vi "Send Serial Command.vi"(7 "Listen for response (T)":bool=TRUE, 8 "error in (no error)":errorcluster, 10 "Command":string, 11 "VISA in":refnum<visa-resource-name>) -> (0 "error out":errorcluster, 2 "Response":string, 3 "VISA out":refnum<visa-resource-name>)   [LabVIEW 2017, in "Drivers.lvlib" / "ASI TG-1000.lvlib"]
doc: "Sends serial command to ASI controller, which should already be configured and initialized."
uses:
  ASI TG-1000.lvlib
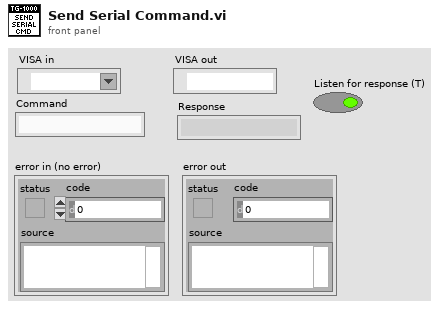
[diagram p1: front panel]
types:
  T1 = typedef "Semaphore RefNum" = refnum<k1>
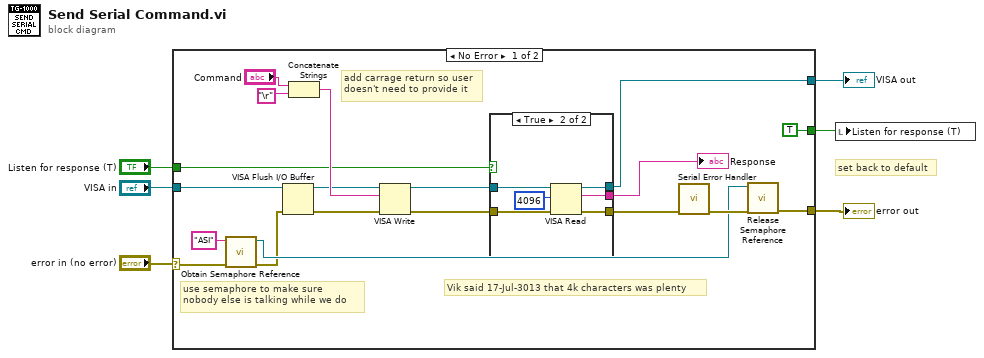
[diagram p0: block diagram]
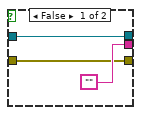
[diagram p2: hidden frame]
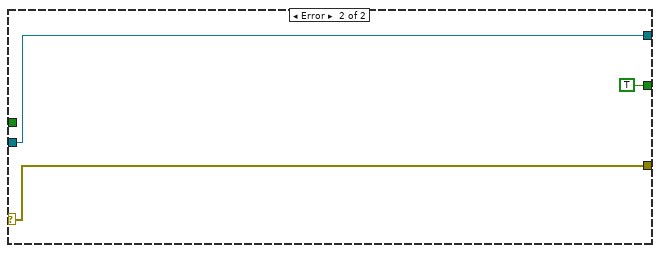
[diagram p3: hidden frame]
diagram:
  # "set back to default"
  n1 = case shown="No Error" "error in (no error)" {
    selector: "error in (no error)" -> [w17 w37]
    tunnel: [w14 w37] -> w6
    tunnel: "VISA in" -> [w11 w36]
    tunnel: [w18 w36] -> w3
    tunnel: "Listen for response (T)" -> [w8 _]
    tunnel: [TRUE TRUE] -> w1
    frame No Error {
      # "use semaphore to make sure\nnobody else is talking while we do"
      # "add carrage return so user\ndoesn't need to provide it"
      # "Vik said 17-Jul-3013 that 4k characters was plenty"
      n2 = call <vilib>:"Obtain Semaphore Reference.vi"("error in (no error)"=w17, "name (unnamed)"="ASI") -> ("error out"=w12:errorcluster, "semaphore"=w13:T1)  [unwired: 3 in, 1 out]
      n3 = VISA Flush I/O Buffer(VISA resource name=w11, error in (no error)=w12) -> (VISA resource name out=w10:refnum<visa-resource-name>, error out=w9:errorcluster)  [unwired: 1 in]
      n4 = Concatenate Strings("Command", "\r") -> (w21:string)
      n5 = VISA Write(VISA resource name=w10, write buffer=w21, error in (no error)=w9) -> (VISA resource name out=w25:refnum<visa-resource-name>, error out=w24:errorcluster)  [unwired: 1 out]
      n6 = case shown="True" w8 {
        tunnel: w25 -> [w26 w34]
        tunnel: w24 -> [w27 w33]
        tunnel: ["" w31] -> w20
        tunnel: [w27 w30] -> w19
        tunnel: [w26 w29] -> w18
        frame False {
        }
        frame True {
          n7 = VISA Read(VISA resource name=w34, byte count=u32 4096, error in (no error)=w33) -> (VISA resource name out=w29:refnum<visa-resource-name>, read buffer=w31:string, error out=w30:errorcluster)  [unwired: 1 out]
        }
      }
      "Response" <- w20
      n8 = call "Serial Error Handler.vi"("error in (no error)"=w19) -> ("error out"=w15:errorcluster)  [unwired: 10 in]
      n9 = call <vilib>:"Release Semaphore Reference.vi"("error in (no error)"=w15, "semaphore"=w13) -> ("error out"=w14:errorcluster)  [unwired: 8 in, 1 out]
    }
    frame Error {
    }
  }
  "error out" <- w6
  "VISA out" <- w3
  n10 = local write "Listen for response (T)"(w1) -> ()
